vi "Scpi_send_test.vi"() -> ()   [LabVIEW 2009]
panel:
  out "size(s)":i32
  out "loops":i32
  in  "Commands":string[](array[string])=["*IDN?", ":SYST:VER\u0000S?", ":SERV:SENS:TYPE?"]
  out "error out":errorcluster
  in  "Instrument":T1(ring)
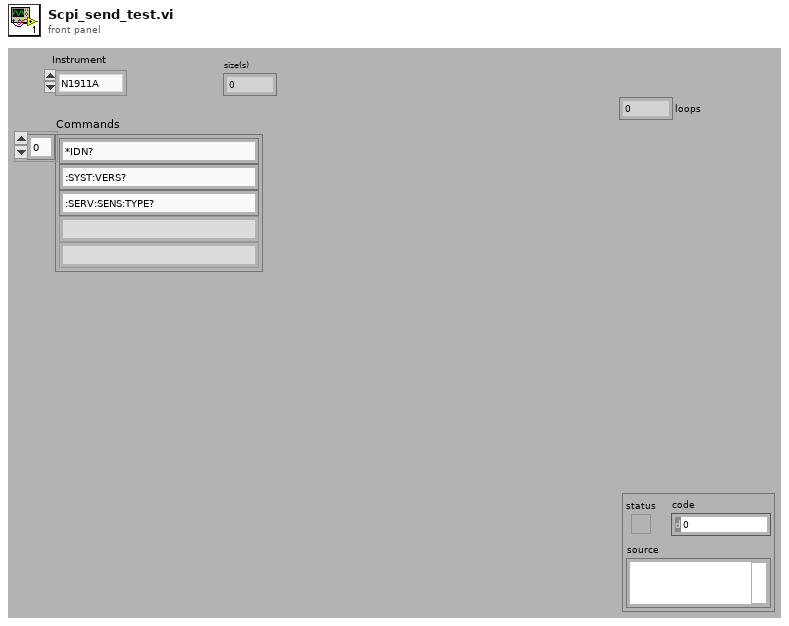
[diagram p1: front panel]
types:
  T1 = enum16{"N1911A", "Siggen", "34980a", "E4418B", "Rvp8"}
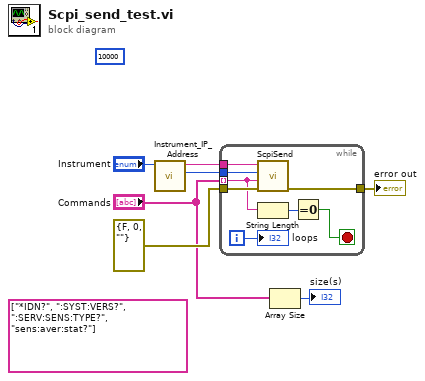
[diagram p0: block diagram]
diagram:
  (unwired) string[] ["*IDN?", ":SYST:VERS?", ":SERV:SENS:TYPE?", "sens:aver:stat?"] ("Commands")
  (unwired) 10000 ("timeout ms (60000)")
  n1 = call "Instrument_IP_Address.vi"("Instrument"="Instrument") -> ("Port"=w5:u16, "IP Address"=w6:string)  [unwired: 9 in]
  n2 = while {
    tunnel: w6 -> [w15]
    tunnel: w5 -> [w14]
    tunnel: "Commands" -> [w11] mode=indexing
    tunnel: errorcluster {"status"=FALSE, "code"=0, "source"=""} ("error in (no error)") -> [w13]
    tunnel: [w12] -> w3
    i -> [w9]
    stop <- w8 stop-if-true
    n3 = call "ScpiSend.vi"("error in (no error)"=w13, "Command"=w11, "TCP port"=w14, "IP Address"=w15) -> ("error out"=w12:errorcluster)  [unwired: 7 in]
    n4 = String Length(string=w11) -> (length=w10:i32)
    n5 = Equal To 0?(x=w10) -> (x = 0?=w8:bool)
    "loops" <- w9
  }
  "error out" <- w3
  n6 = Array Size(array="Commands") -> (size(s)=→"size(s)":i32)
